vi "DLConnect-Com-Exec.vi"(8 "error in (no error)":errorcluster, 9 "ControlQueue":refnum<queue>, 10 "data":variant, 11 "DelayLine in":refnum<class "DelayLine.lvclass">) -> (0 "error out":errorcluster, 3 "DelayLine out":refnum<class "DelayLine.lvclass">)   [LabVIEW 2020, in "DelayLine.lvclass"]
uses:
  DelayLine.lvclass
  C:/dev/TRANCON/Classes/GeneralFunctionality/GeneralFunctionality.lvclass
  dependecies/ControlsVIs/Clusters-def/DL-Reply-to-Connect-to-Client.ctl
  dependecies/ControlsVIs/Clusters-def/SERVER-Commands.ctl
  dependecies/ControlsVIs/Clusters-def/DL-Reply-to-Connect.ctl
  GeneralFunctionality/GeneralFunctionality.lvclass/GeneralFunctionality.ctl
  Control/Control-Server/Control-Server.lvclass
  GeneralFunctionality/GeneralFunctionality.lvclass
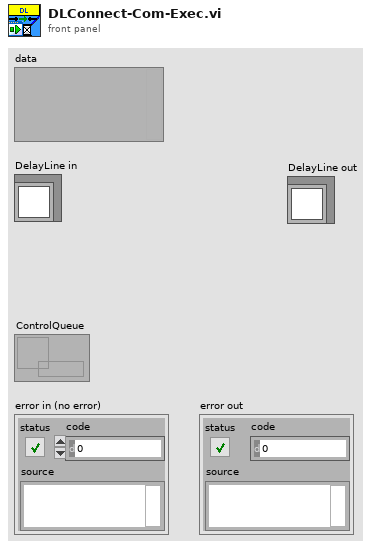
[diagram p1: front panel]
types:
  T1 = typedef "Control-Server.lvclass/SERVER-Commands.ctl" = string
  T2 = typedef "DelayLine.lvclass/DL-Reply-to-Connect.ctl" = cluster{"On/Off":bool, "error":errorcluster, "DelayLine.lvclass":refnum<class "DelayLine.lvclass">}
  T3 = typedef "DelayLine.lvclass/DL-Reply-to-Connect-to-Client.ctl" = cluster{"on/off":bool, "pos":dbl[], "param":cluster{"min":dbl, "max":dbl, "real pos":dbl}[], "predefine_pos":dbl[][], "error":errorcluster}
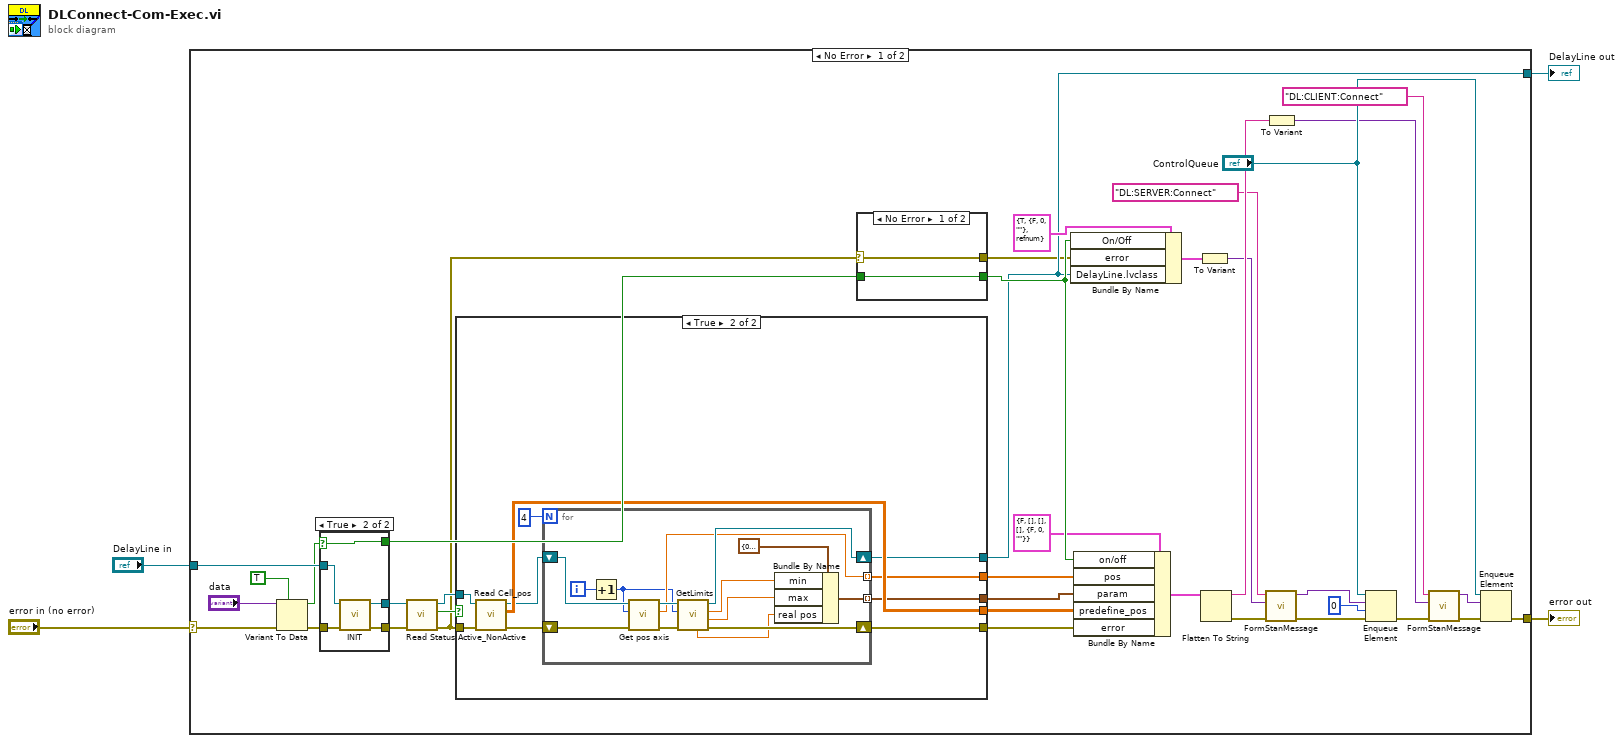
[diagram p0: block diagram]
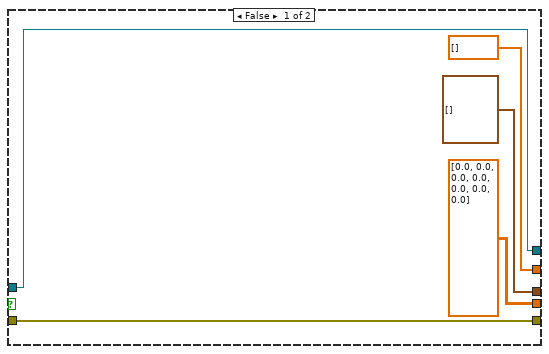
[diagram p2: hidden frame]
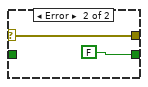
[diagram p3: hidden frame]
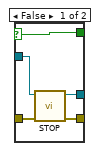
[diagram p4: hidden frame]
diagram:
  n1 = case shown="No Error" "error in (no error)" {
    selector: "error in (no error)" -> [w29 w86]
    tunnel: "DelayLine in" -> [w41 w85]
    tunnel: [w18 w86] -> w3
    tunnel: [w10 w85] -> w2
    frame No Error {
      n2 = Variant To Data(error in=w29, type=TRUE, Variant="data") -> (data=w32:bool, error out=w33:errorcluster)
      n3 = case shown="True" w32 {
        selector: w32 -> [w76 w81]
        tunnel: [w79 w82] -> w28
        tunnel: [w78 w83] -> w26
        tunnel: w33 -> [w77 w84]
        tunnel: [w76 w81] -> w34
        tunnel: w41 -> [w75 w80]
        frame False {
          n4 = call-dynamic "STOP.vi"("error in (no error)"=w77, "Stop in"=w75) -> ("error out"=w78:errorcluster, "Stop out"=w79:refnum<class "DelayLine.lvclass">)  [unwired: 8 in]
        }
        frame True {
          n5 = call-dynamic "INIT.vi"("error in (no error)"=w84, "GeneralFunctionality in"=w80) -> ("error out"=w83:errorcluster, "GeneralFunctionality out"=w82:refnum<class "DelayLine.lvclass">)  [unwired: 8 in]
        }
      }
      n6 = call "Read Status Active_NonActive.vi"("error in (no error)"=w26, "GeneralFunctionality in"=w28) -> ("error out"=w5:errorcluster, "Status Active/NonActive"=w27:bool, "GeneralFunctionality out"=w11:refnum<class "DelayLine.lvclass">)  [unwired: 7 in]
      n7 = case shown="True" w27 {
        tunnel: w11 -> [w44 w55]
        tunnel: w5 -> [w46 w53]
        tunnel: [w46 w49] -> w6
        tunnel: [dbl[][] [[0.0, 0.0, 0.0, 0.0, 0.0, 0.0, 0.0]] ("Cell_pos") w56] -> w12
        tunnel: [w44 w50] -> w10
        tunnel: [dbl[] [] w48] -> w9
        tunnel: [cluster{"min":dbl, "max":dbl, "real pos":dbl}[] [] w47] -> w8
        frame False {
        }
        frame True {
          n8 = call "Read Cell_pos.vi"("error in (no error)"=w53, "DelayLine in"=w55) -> ("error out"=w51:errorcluster, "Cell_pos"=w56:dbl[][], "DelayLine out"=w52:refnum<class "DelayLine.lvclass">)  [unwired: 7 in]
          n9 = for {
            N: 4 -> [_]
            shift-right: [w67] -> w50
            shift-left: w52 -> [w66]
            shift-right: [w64] -> w49
            shift-left: w51 -> [w65]
            tunnel: [w63] -> w48 mode=indexing
            tunnel: [w58] -> w47 mode=indexing
            i -> [w70]
            n10 = Increment(x=w70) -> (x+1=w57:i32)
            n11 = call-dynamic "Get pos axis.vi"("error in (no error)"=w65, "Axis"=w57, "DelayLine in"=w66) -> ("error out"=w69:errorcluster, "Pos"=w63:dbl, "DelayLine out"=w68:refnum<class "DelayLine.lvclass">)  [unwired: 6 in]
            n12 = call-dynamic "GetLimits.vi"("error in (no error)"=w69, "Axis"=w57, "DelayLine in"=w68) -> ("error out"=w64:errorcluster, "max"=w60:dbl, "min"=w61:dbl, "DelayLine out"=w67:refnum<class "DelayLine.lvclass">, "real pos, mm"=w59:dbl)  [unwired: 4 in]
            n13 = Bundle By Name(cluster=cluster{"min":dbl, "max":dbl, "real pos":dbl} {"min"=0.0, "max"=0.0, "real pos"=0.0} ("axis"), "min"=w61, "max"=w60, "real pos"=w59) -> (w58:cluster{"min":dbl, "max":dbl, "real pos":dbl})
          }
        }
      }
      n14 = case shown="No Error" w5 {
        selector: w5 -> [w71 w73]
        tunnel: [w72 FALSE] -> w40
        tunnel: w34 -> [w72 _]
        tunnel: [w71 w73] -> w7
        frame No Error {
        }
        frame Error {
        }
      }
      n15 = Bundle By Name(cluster=T2 {"On/Off"=TRUE, "error"={"status"=FALSE, "code"=0, "source"=""}, "DelayLine.lvclass"=refnum}, "On/Off"=w40, "error"=w7, "DelayLine.lvclass"=w10) -> (w39:T2)
      n16 = Bundle By Name(cluster=T3 {"on/off"=FALSE, "pos"=[], "param"=[], "predefine_pos"=[], "error"={"status"=FALSE, "code"=0, "source"=""}} ("output cluster"), "on/off"=w40, "pos"=w9, "param"=w8, "predefine_pos"=w12, "error"=w6) -> (w36:T3)
      n17 = To Variant(anything=w39) -> (Variant=w14:variant)
      n18 = Flatten To String(anything=w36) -> (data string=w37:string, error out=w24:errorcluster)  [unwired: 3 in, 1 out]
      n19 = call "FormStanMessage.vi"("error in"=w24, "data"=w14, "Command"=T1 "DL:SERVER:Connect" ("Commands")) -> ("error out"=w23:errorcluster, "message"=w22:variant)  [unwired: 7 in]
      n20 = To Variant(anything=w37) -> (Variant=w13:variant)
      n21 = Enqueue Element(queue="ControlQueue", element=w22, timeout in ms (-1)=0, error in (no error)=w23) -> (error out=w20:errorcluster)  [unwired: 2 out]
      n22 = call "FormStanMessage.vi"("error in"=w20, "data"=w13, "Command"=T1 "DL:CLIENT:Connect" ("Commands")) -> ("error out"=w19:errorcluster, "message"=w16:variant)  [unwired: 7 in]
      n23 = Enqueue Element(queue="ControlQueue", element=w16, error in (no error)=w19) -> (error out=w18:errorcluster)  [unwired: 1 in, 2 out]
    }
    frame Error {
    }
  }
  "DelayLine out" <- w2
  "error out" <- w3
